vi "gen_rng block.vi"() -> (1 "display arr":u8[][](array[numeric]), 3 "Random block":u8[](array[numeric]))   [LabVIEW 2024]
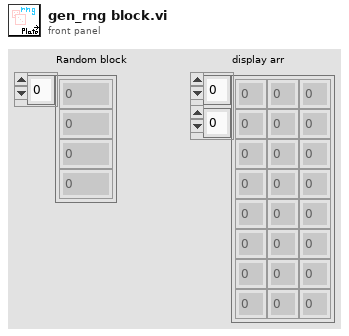
[diagram p1: front panel]
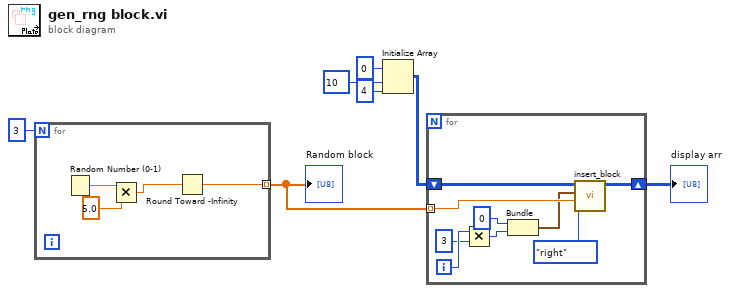
[diagram p0: block diagram]
diagram:
  n1 = for {
    N: 3 -> [_]
    tunnel: [w8] -> w6 mode=indexing
    n2 = Random Number (0-1)() -> (number: 0 to 1=w11:dbl)
    n3 = Multiply(x=w11, y=5.0) -> (x*y=w9:dbl)
    n4 = Round Toward -Infinity(1:w9) -> (0:w8:dbl)
  }
  "Random block" <- w6
  n5 = Initialize Array(u8 0 ("element"), 10 ("dimension size"), 4 ("dimension size")) -> (w2:u8[][])
  n6 = for {
    tunnel: w6 -> [w20] mode=indexing
    shift-right: [w14] -> w1
    shift-left: w2 -> [w15]
    i -> [w19]
    n7 = Multiply(x=w19, y=3) -> (x*y=w13:i32)
    n8 = Bundle(0, w13) -> (w17:cluster{i32, i32})  [unwired: 1 in]
    n9 = call "insert_block.vi"("direction"=enum16{"up", "right", "down", "left"}."right", "block_type"=w20, "position"=w17, "plate arr"=w15) -> ("return plate"=w14:u8[][])  [unwired: 6 in, 1 out]
  }
  "display arr" <- w1
